vi "getDelay.vi"(8 "error in (no error)":errorcluster, 11 "Instrument.DelayLine in":refnum<class "Instrument.DelayLine.lvclass">) -> (0 "error out":errorcluster, 2 "delay (ps)":dbl, 3 "Instrument.DelayLine out":refnum<class "Instrument.DelayLine.lvclass">, 4 "Finished?":bool)   [LabVIEW 2019, in "Instrument.DelayLine.lvclass"]
uses:
  Instrument.DelayLine.lvclass
  Typedefs/DelayLine.Commands--Enum.ctl
  Typedefs/DelayLine.getDelay--cluster.ctl
  0169b2a0-9071-4ecc-bbd0-17af7c548e9a.vi
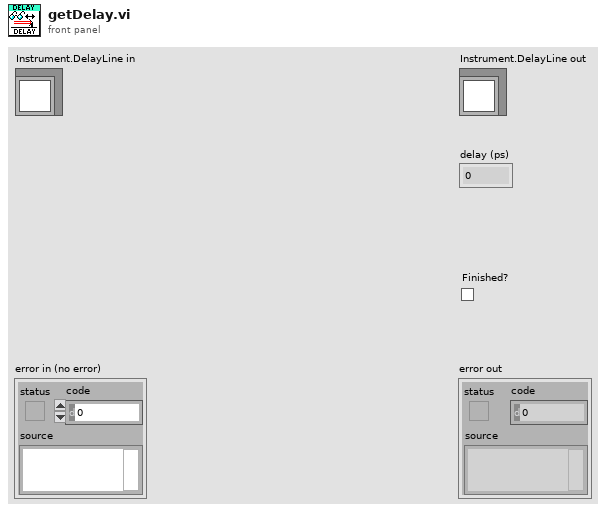
[diagram p1: front panel]
types:
  T1 = typedef "Instrument.DelayLine.lvclass/DelayLine.getDelay--cluster.ctl" = cluster{"delay":dbl, "Finished?":bool}
  T2 = typedef "Instrument.DelayLine.lvclass/DelayLine.Commands--Enum.ctl" = enum16{"getDelay", "setDelay"}
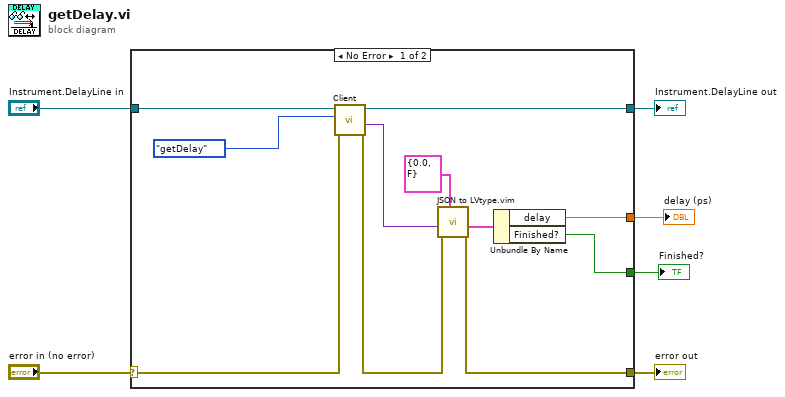
[diagram p0: block diagram]
diagram:
  n1 = case shown="No Error" "error in (no error)" {
    selector: "error in (no error)" -> [w14 w19]
    tunnel: [w12 w19] -> w5
    tunnel: [w17 w18] -> w3
    tunnel: "Instrument.DelayLine in" -> [w16 w18]
    tunnel: [w8 _] -> w2
    tunnel: [w7 _] -> w1
    frame No Error {
      n2 = call-dynamic "Client.vi"("error in (no error)"=w14, "Command in"=DelayLine.Commands--Enum."getDelay" ("command"), "Instrument in"=w16) -> ("error out"=w13:errorcluster, "Data out"=w11:variant, "Instrument out"=w17:refnum<class "Instrument.DelayLine.lvclass">)  [unwired: 5 in, 1 out]
      n3 = call "JSON to LVtype.vim"("type"=T1 {"delay"=0.0, "Finished?"=FALSE} ("getDelay"), "error in (no error)"=w13, "JSON Data in"=w11) -> ("error out"=w12:errorcluster, "Data out"=w9:T1)  [unwired: 7 in]
      n4 = Unbundle By Name(w9) -> ("delay"=w8:dbl, "Finished?"=w7:bool)
    }
    frame Error {
    }
  }
  "error out" <- w5
  "Instrument.DelayLine out" <- w3
  "delay (ps)" <- w2
  "Finished?" <- w1
